vi "Robot Global Data.vi"() -> ()   [LabVIEW 2016]
doc: "This global VI can contain as many global variables as you need. Place a control on the panel, give it a good name. To read or write to it from a VI, drag the icon to the diagram of that VI. You can also drag from the project. Click on the node to change which global you access. You shouldn't have multiple locations writing to a global or it will cause a race-condition."
uses:
  <vilib>/Rock Robotics/WPI/Camera/WPI_CameraImageSize.ctl
  <vilib>/Rock Robotics/WPI/DriverStation/WPI_DriverStationRobotMode2.ctl
panel:
  in  "Pi Vision":string
  in  "Controller 1":T1
  in  "Teleop Called Times?":dbl=3318.0
  in  "Stop Periodic Tasks Logging":bool
  out "FMS Attached?":bool
  in  "Vision Server":T2
  in  "ADB TCP Port":u16=3061
  in  "Items Written":dbl=3030.0
  in  "Items Enqueued":dbl=3030.0
  in  "Forward Headings":dbl[](array[numeric])=[3816.0, 462.0, 2262.0, 388.0]
  in  "Setpoint 4":dbl=-2048.0
  in  "Setpoint 3":dbl=6144.0
  in  "Setpoint 2":dbl
  in  "Setpoint 1":dbl
  in  "Wheel Speed":T3
  in  "Swerve Speed":T4
  in  "Encoder Offsets":T5={"Encoder Offset 1"=16, "Encoder Offset 2"=-36, "Encoder Offset 3"=6156, "Encoder Offset 4"=-2024}
  in  "Robot Mode":T6=enum."Finish"
  in  "image size":T7=enum."320x240"
  in  "Enable Vision":bool
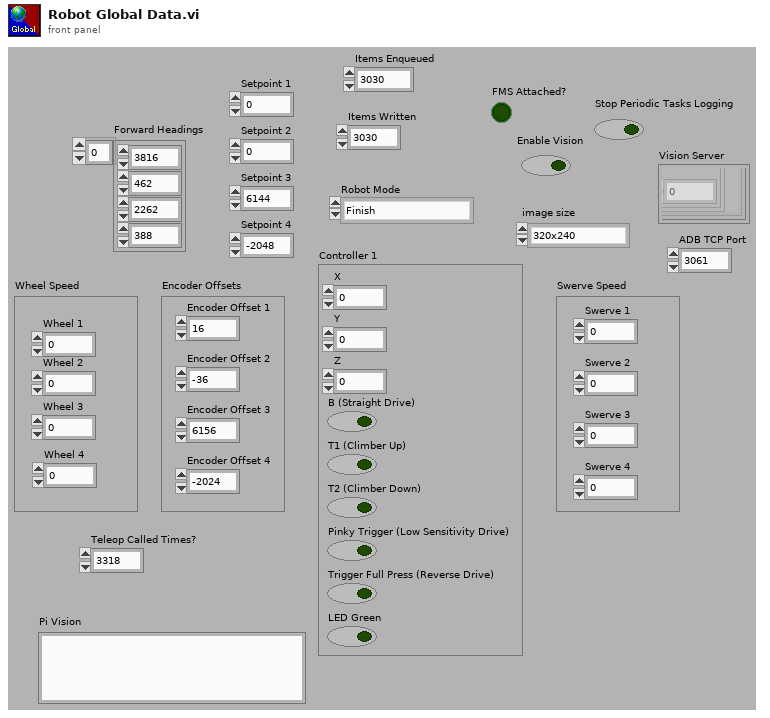
[diagram p1: front panel]
types:
  T1 = cluster{"X":dbl, "Y":dbl, "Z":dbl, "B (Straight Drive)":bool, "T1 (Climber Up)":bool, "T2 (Climber Down)":bool, "Pinky Trigger (Low Sensitivity Drive)":bool, "Trigger Full Press (Reverse Drive)":bool, "LED Green":bool}
  T2 = cluster{"connection ID":refnum<k5>, "Running?":bool, "TCP Port":u16, "LastMessageReceivedTime":dbl, "WantsAppRestart":bool, "IsConnect":bool, "Vision Updates":cluster{"CapturedAgoMs":i32, "Valid?":bool, "CapturedAtTimestamp":dbl, "Targets":cluster{"X":dbl, "Y":dbl, "Z":dbl}[]}[]}
  T3 = cluster{"Wheel 1":dbl, "Wheel 2":dbl, "Wheel 3":dbl, "Wheel 4":dbl}
  T4 = cluster{"Swerve 1":dbl, "Swerve 2":dbl, "Swerve 3":dbl, "Swerve 4":dbl}
  T5 = cluster{"Encoder Offset 1":i32, "Encoder Offset 2":i32, "Encoder Offset 3":i32, "Encoder Offset 4":i32}
  T6 = typedef "WPI_DriverStationRobotMode2.ctl" = enum16{"Autonomous Disabled", "Autonomous Enabled", "Teleop Disabled", "Teleop Enabled", "Disconnected", "Finish", "Test Disabled", "Test Enabled", "Emergency Stopped"}
  T7 = typedef "WPI_CameraImageSize.ctl" = enum16{"640x480", "320x240", "160x120", "Custom"}
diagram:
